vi "Gui_SetupData.vi"(8 "error in (no error)":errorcluster, 11 "Variant":variant) -> (0 "error out":errorcluster caption="sortie d'erreur", 3 "Variant out":variant)   [LabVIEW 2017]
uses:
  controls/DATA_Inputs.ctl
  controls/SEQUENCE_Inputs.ctl
  controls/TRAPPING_Inputs.ctl
  controls/EXCIT_Inputs.ctl
  controls/TIMING_Inputs.ctl
  controls/PROCESSING_Inputs.ctl
panel:
  in  "Vertical Range (pk-pk)":dbl(ring)=10.0 caption="Sample Rate" items=["0.2"=0.2, "0.4"=0.4, "1"=1.0, "2"=2.0, "4"=4.0, "10"=10.0]
  in  "OK":bool
  out "Number Of Acquisitions":i16
  out "DATA Inputs":T1={"Record Length"=100000, "Sample Rate"=10000000.0, "Data Type"=0, "Vertical Range"=10.0, "Acquisition Duration"=100000.0} {"Vertical Range" items=["0.2"=0.2, "0.4"=0.4, "1"=1.0, "2"=2.0, "4"=4.0, "10"=10.0]; "Data Type" items=["I16", "DBL"]; "Sample Rate" items=["1 MHz"=1000000.0, "2 MHz"=2000000.0, "5 MHz"=5000000.0, "10 MHz"=10000000.0, "20 MHz"=20000000.0, "25 MHz"=25000000.0, "50 MHz"=50000000.0, "100 MHz"=100000000.0]}
  in  "Sample Rate":dbl(ring)=10000000.0 items=["1 MHz"=1000000.0, "2 MHz"=2000000.0, "5 MHz"=5000000.0, "10 MHz"=10000000.0, "20 MHz"=20000000.0, "25 MHz"=25000000.0, "50 MHz"=50000000.0, "100 MHz"=100000000.0]
  in  "Acquisition Duration (ms)":dbl
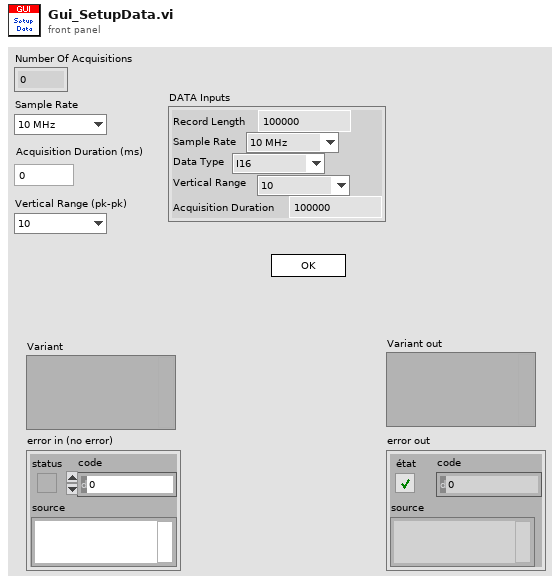
[diagram p1: front panel]
types:
  T1 = typedef "DATA_Inputs.ctl" = cluster{"Record Length":i32, "Sample Rate":dbl, "Data Type":u8, "Vertical Range":dbl, "Acquisition Duration":dbl}
  T2 = typedef "SEQUENCE_Inputs.ctl" = cluster{"TRAPPING Inputs":T3, "EXCIT Inputs":T4, "DATA Inputs":T1, "TIMING Inputs":T5, "PROCESSING  Inputs":T6}
  T3 = typedef "TRAPPING_Inputs.ctl" = cluster{"Number of Channels":i32, "Init Values":dbl[], "Opening Values":dbl[], "Trapping Values":dbl[], "Emptying Values":dbl[], "Adiabatic ON":bool, "Adiabatic Duration":i32, "Adiabatic Waveforms":string[]}
  T4 = typedef "EXCIT_Inputs.ctl" = cluster{"Number of Excitations":i32, "Script Text":string, "Table of Waveforms":string[]}
  T5 = typedef "TIMING_Inputs.ctl" = cluster{"Number of Acquisitions ":i16, "Number of Accumulations":i16, "Table of Waveforms":string[], "Script Text":string}
  T6 = typedef "PROCESSING_Inputs.ctl" = cluster{"Reference Mass":dbl, "Cyclotron Freq":dbl, "Magnetron Freq":dbl}
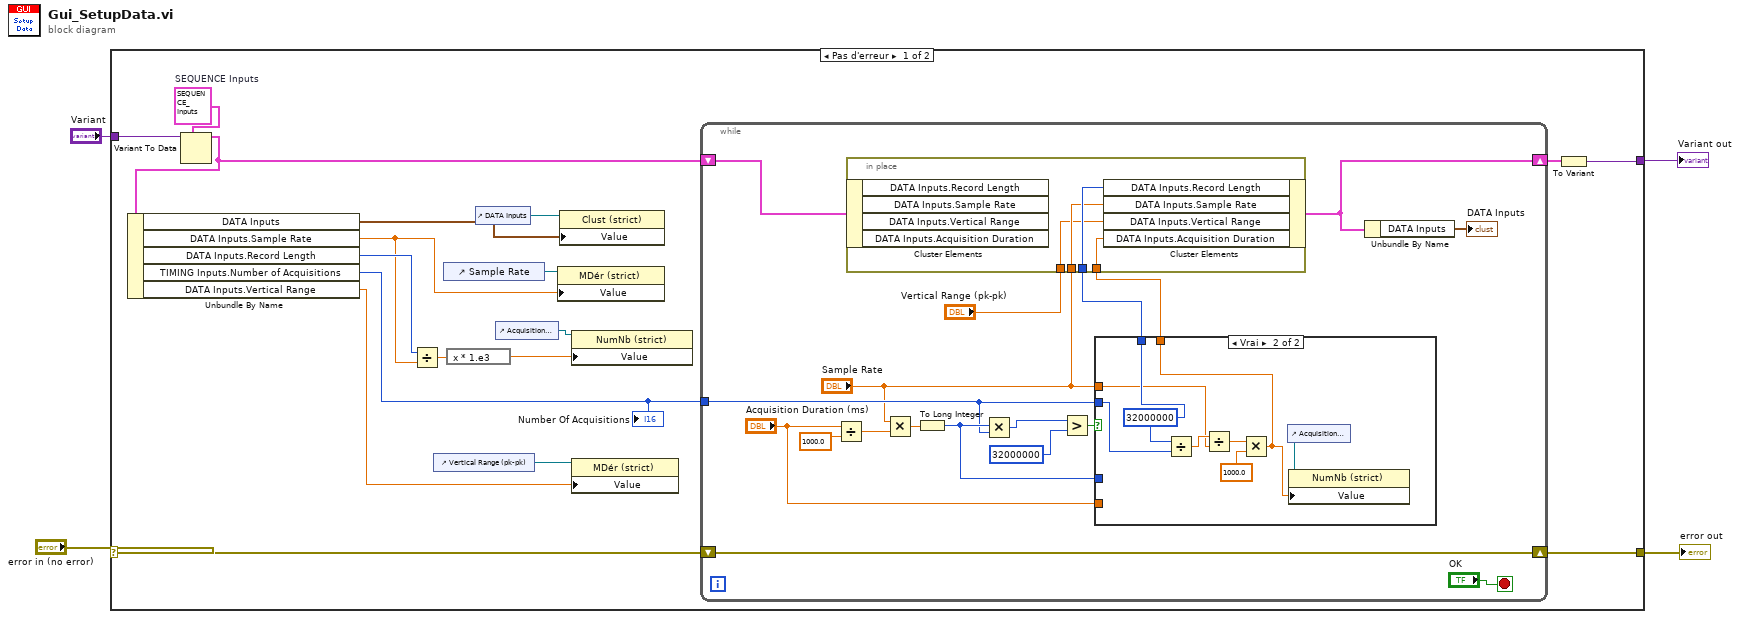
[diagram p0: block diagram]
diagram:
  n1 = case shown="Pas d'erreur" "error in (no error)" {
    selector: "error in (no error)" -> [w22 w56]
    tunnel: [w21 w56] -> w3
    tunnel: "Variant" -> [w19 w55]
    tunnel: [w9 w55] -> w1
    frame No Error {
      w20 = T2 {"TRAPPING Inputs"={"Number of Channels"=4, "Init Values"=[2.0, 5.0, 5.0, 2.0], "Opening Values"=[0.0, 0.0, 0.0, 0.0], "Trapping Values"=[2.0, 5.0, 5.0, 2.0], "Emptying Values"=[-5.0, -5.0, -5.0, -5.0], "Adiabatic ON"=FALSE, "Adiabatic Duration"=0, "Adiabatic Waveforms"=["Adiabatic_None_2_2_2000.bin", "Adiabatic_Ramp_5_0_2000.bin", "Adiabatic_DoubleRamp_5_0_2000.bin", "Adiabatic_RC_2_0_2000.bin"]}, "EXCIT Inputs"={"Number of Excitations"=1, "Script Text"="", "Table of Waveforms"=[]}, "DATA Inputs"={"Record Length"=8192, "Sample Rate"=4.0, "Data Type"=0, "Vertical Range"=0.0, "Acquisition Duration"=100000.0}, "TIMING Inputs"={"Number of Acquisitions "=1, "Number of Accumulations"=1, "Table of Waveforms"=[], "Script Text"=""}, "PROCESSING  Inputs"={"Reference Mass"=300.0939, "Cyclotron Freq"=255.727, "Magnetron Freq"=0.001}}  # SEQUENCE Inputs
      n2 = Variant To Data(type=w20, Variant=w19) -> (data=w18:T2)  [unwired: 1 in, 1 out]
      n3 = Unbundle By Name(w18) -> ("DATA Inputs"=w12:T1, "DATA Inputs.Sample Rate"=w13:dbl, "DATA Inputs.Record Length"=w15:i32, "TIMING Inputs.Number of Acquisitions"=w7:i16, "DATA Inputs.Vertical Range"=w5:dbl)
      "Number Of Acquisitions" <- w7
      n4 = Divide(x=w15, y=w13) -> (x/y=w14:dbl)
      n5 = control-ref of="Vertical Range (pk-pk)"() -> (w6:refnum<vi>)
      n6 = control-ref of="Sample Rate"() -> (w17:refnum<vi>)
      n7 = expression code="x * 1.e3"(w14) -> (w16:dbl)
      n8 = control-ref of="DATA Inputs"() -> (w8:refnum<vi>)
      n9 = control-ref of="Acquisition Duration (ms)"() -> (w11:refnum<vi>)
      n10 = property class="MDér (strict)"(reference=w17, "Value"=w13) -> ()  [unwired: 1 in, 2 out]
      n11 = property class="Clust (strict)"(reference=w8, "Value"=w12) -> ()  [unwired: 1 in, 2 out]
      n12 = property class="NumNb (strict)"(reference=w11, "Value"=w16) -> ()  [unwired: 1 in, 2 out]
      n13 = property class="MDér (strict)"(reference=w6, "Value"=w5) -> ()  [unwired: 1 in, 2 out]
      n14 = while {
        shift-right: [w40] -> w21
        shift-left: w22 -> [w40]
        shift-right: [w27] -> w10
        shift-left: w18 -> [w39]
        tunnel: w7 -> [w32]
        stop <- "OK" stop-if-true
        n15 = Divide(x="Acquisition Duration (ms)", y=1000.0) -> (x/y=w38:dbl)
        n16 = Multiply(x="Sample Rate", y=w38) -> (x*y=w37:dbl)
        n17 = To Long Integer(number=w37) -> (32bit integer=w33:i32)
        n18 = Multiply(x=w33, y=w32) -> (x*y=w35:i32)
        n19 = Greater?(x=w35, y=32000000) -> (0:w36:bool)
        n20 = case shown="Vrai" w36 {
          tunnel: "Sample Rate" -> [_ w49]
          tunnel: w32 -> [_ w54]
          tunnel: [w46 w50] -> w31
          tunnel: w33 -> [w46 _]
          tunnel: "Acquisition Duration (ms)" -> [w45 _]
          tunnel: [w45 w47] -> w23
          frame False {
          }
          frame True {
            w50 = 32000000 ("x")
            n21 = Divide(x=w50, y=w54) -> (x/y=w53:dbl)
            n22 = Divide(x=w53, y=w49) -> (x/y=w52:dbl)
            n23 = Multiply(x=w52, y=1000.0) -> (x*y=w47:dbl)
            n24 = control-ref of="Acquisition Duration (ms)"() -> (w48:refnum<vi>)
            n25 = property class="NumNb (strict)"(reference=w48, "Value"=w47) -> ()  [unwired: 1 in, 2 out]
          }
        }
        n26 = in-place {
          in-place-border: w31 -> [w44]
          in-place-border: "Sample Rate" -> [w43]
          in-place-border: "Vertical Range (pk-pk)" -> [w42]
          in-place-border: w23 -> [w41]
          n27 = in-place-cluster #1(w39) -> ()  [unwired: 4 out]
          n28 = in-place-cluster #1("DATA Inputs.Record Length"=w44, "DATA Inputs.Sample Rate"=w43, "DATA Inputs.Vertical Range"=w42, "DATA Inputs.Acquisition Duration"=w41) -> (w27:T2)
        }
        n29 = Unbundle By Name(w27) -> ("DATA Inputs"=→"DATA Inputs":T1)
      }
      n30 = To Variant(anything=w10) -> (Variant=w9:variant)
    }
    frame Error {
    }
  }
  "error out" <- w3
  "Variant out" <- w1
